vi "ViperHawk Get Diagnostic Data.vi"(6 "Command":enum16{"9E", "9F"}(ring), 10 "Hex String In":string, 11 "Diagnostic":T1) -> (3 "Diagnostic Data Output":T1)   [LabVIEW 2016]
uses:
  Type Definitions/ViperHawk/ViperHawk Diagnostic Data.ctl
  Utility/LabVIEW GEA2 Toolkit v1.0.0.0/library/GEA2_Toolkit.lvlib
  <vilib>/ptbypt/NI_PtbyPt.lvlib
panel:
  out "String":string
  out "Cycle Number":u32
  out "Hex Array Out":u8[](array[numeric]) format="%.0x"
  # "00 00 BF 27 01 B7 00 7B 00 00 00 00 00 00 00 00 14 64 0F 01 01 00 00 81"
  # "9F\n01 02"
  # "9F"
  # "01 02 03 63 00 00 04 00 04 05 00 04 02 00 00 00 00 00 00 00 00 01 00 00 00 00"
  # "9E"
  # "00 00 AA E1 03 65 03 E1 00 00 00 00 00 00 00 00 14 64 0F 01 04 00 00 40"
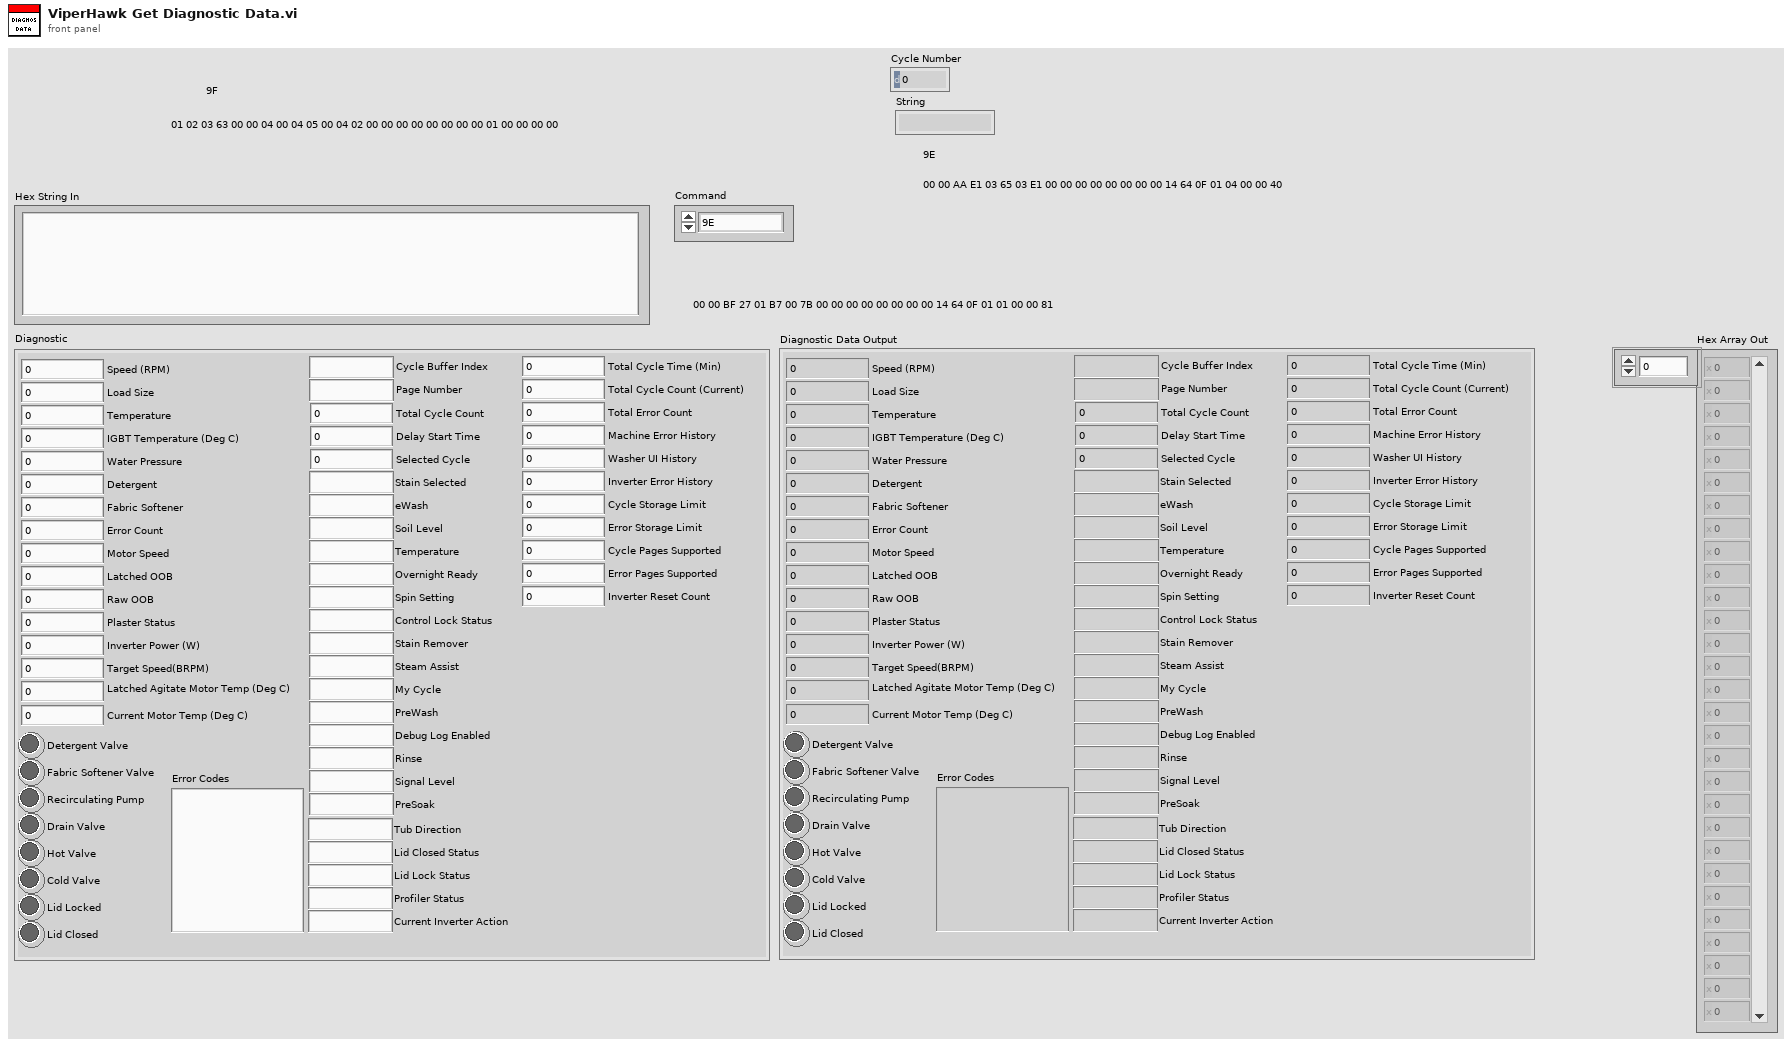
[diagram p1: front panel]
types:
  T1 = typedef "ViperHawk Diagnostic Data.ctl" = cluster{"Speed (RPM)":u32, "Load Size":u32, "Temperature":u32, "Water Pressure":dbl, "Detergent":u32, "Fabric Softener":u32, "Tub Direction":string, "Detergent Valve":bool, "Fabric Softener Valve":bool, "Recirculating Pump":bool, "Drain Valve":bool, "Hot Valve":bool, "Cold Valve":bool, "Lid Closed Status":string, "Lid Lock Status":string, "Error Count":u32, "IGBT Temperature (Deg C)":u32, "Motor Speed":u32, "Latched OOB":u32, "Raw OOB":u32, "Plaster Status":u32, "Inverter Power (W)":u32, "Target Speed(BRPM)":u32, "Latched Agitate Motor Temp (Deg C)":u32, "Current Motor Temp (Deg C)":u32, "Profiler Status":string, "Current Inverter Action":string, "Error Codes":string, "Lid Locked":bool, "Lid Closed":bool, "9E Diagnostic Data":cluster{"Total Cycle Time (Min)":u32, "Total Cycle Count (Current)":u16, "Total Error Count":u16, "Machine Error History":u32, "Washer UI History":u32, "Inverter Error History":u32, "Cycle Storage Limit":u8, "Error Storage Limit":u8, "Cycle Pages Supported":u8, "Error Pages Supported":u8, "Inverter Reset Count":u16}, "9F Diagnostic Data":cluster{"Cycle Buffer Index":string, "Page Number":string, "Total Cycle Count":u32, "Delay Start Time":u32, "Stain Selected":string, "Selected Cycle":u32, "eWash":string, "Soil Level":string, "Temperature":string, "Overnight Ready":string, "Spin Setting":string, "Control Lock Status":string, "Stain Remover":string, "Steam Assist":string, "My Cycle":string, "PreWash":string, "Debug Log Enabled":string, "Rinse":string, "Signal Level":string, "PreSoak":string}}
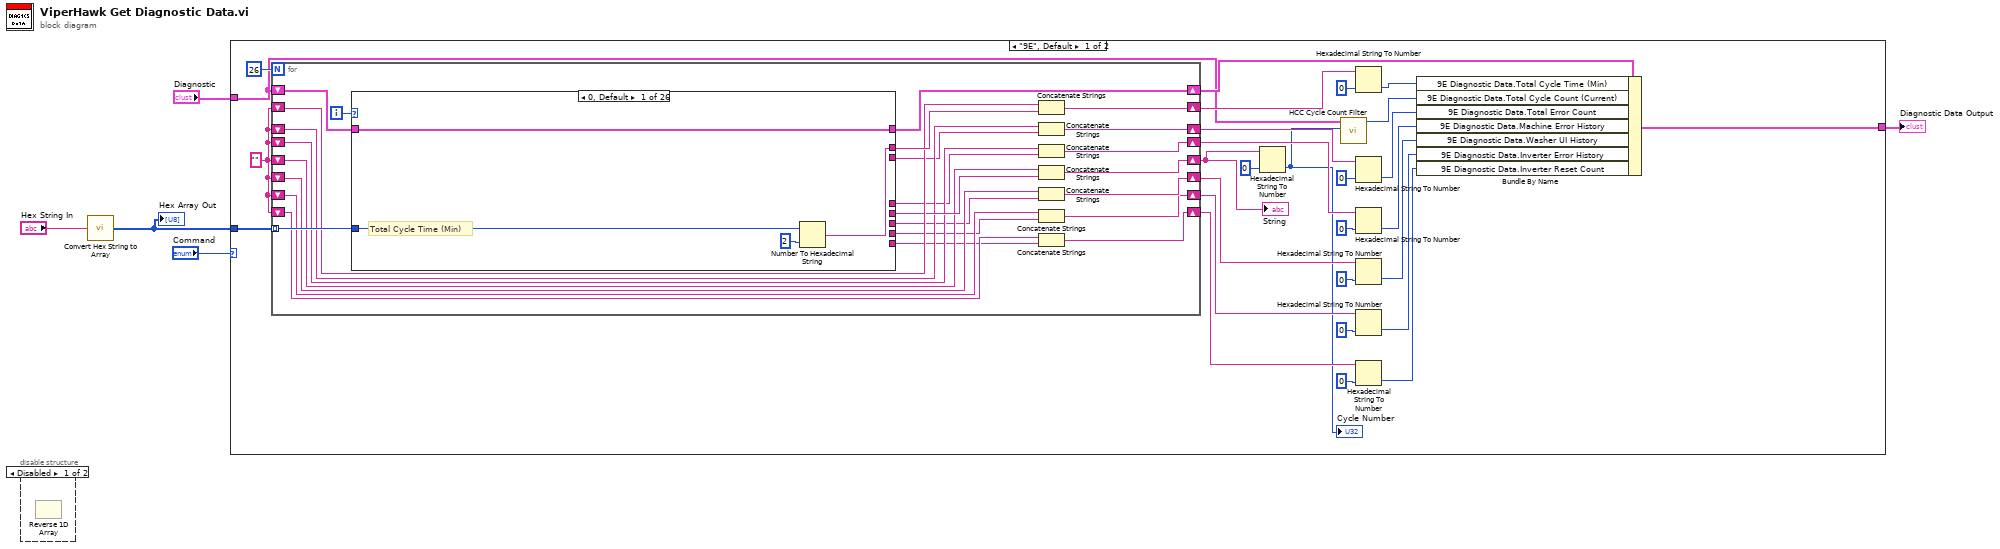
[diagram p0: block diagram]
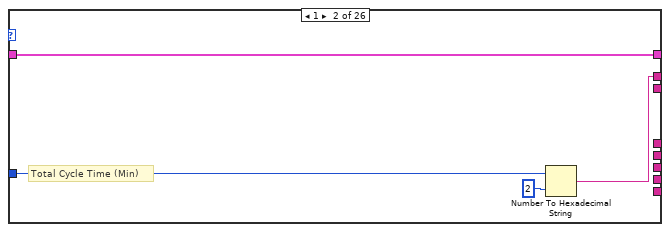
[diagram p3: hidden frame]
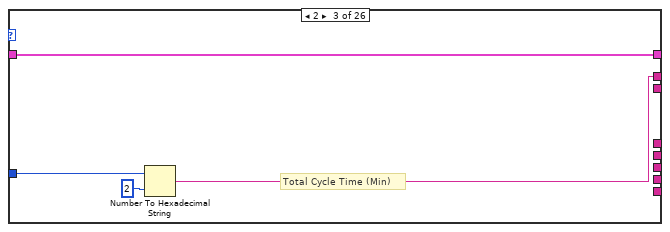
[diagram p4: hidden frame]
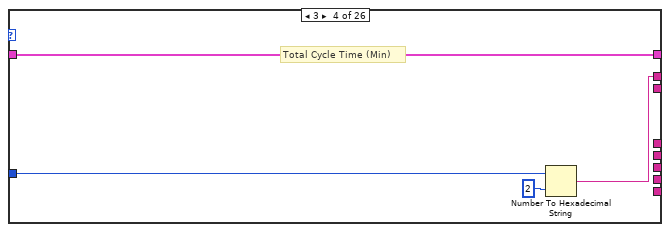
[diagram p5: hidden frame]
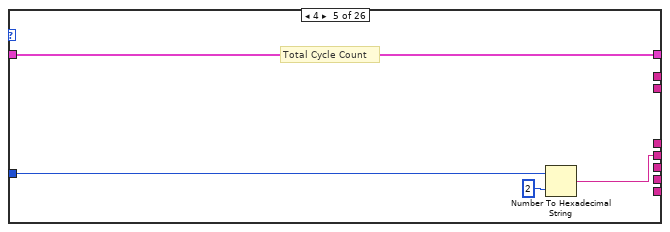
[diagram p6: hidden frame]
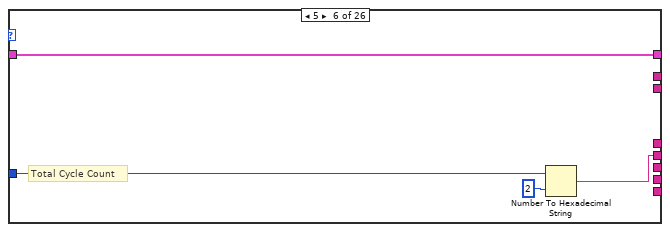
[diagram p7: hidden frame]
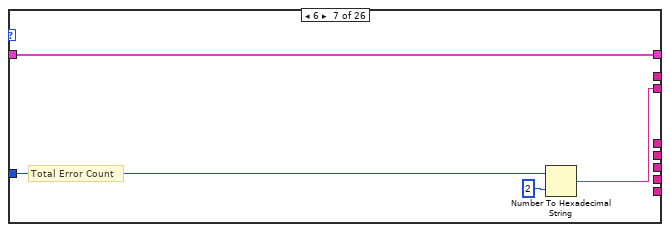
[diagram p8: hidden frame]
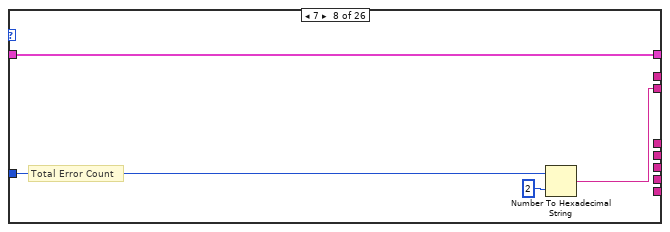
[diagram p9: hidden frame]
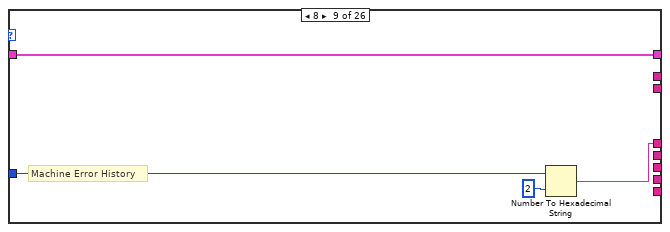
[diagram p10: hidden frame]
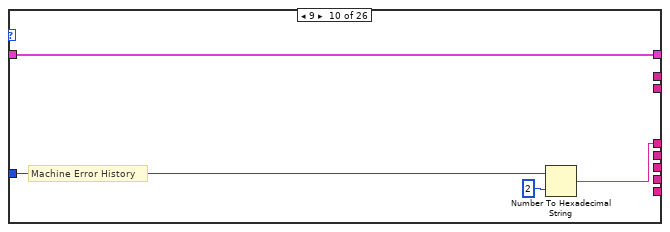
[diagram p11: hidden frame]
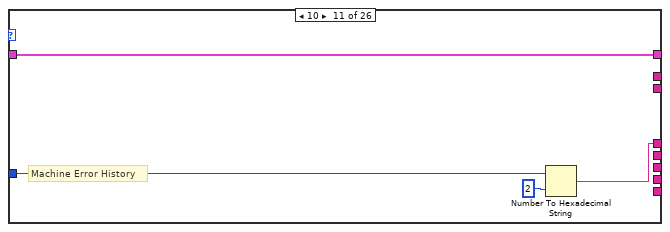
[diagram p12: hidden frame]
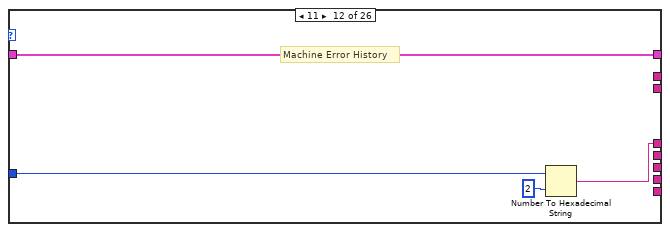
[diagram p13: hidden frame]
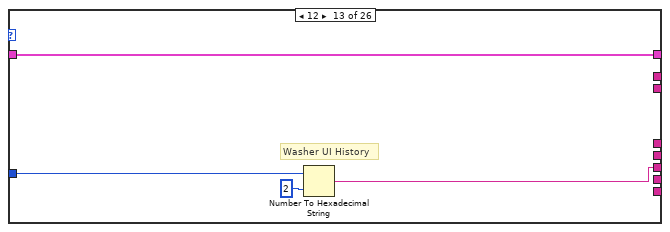
[diagram p14: hidden frame]
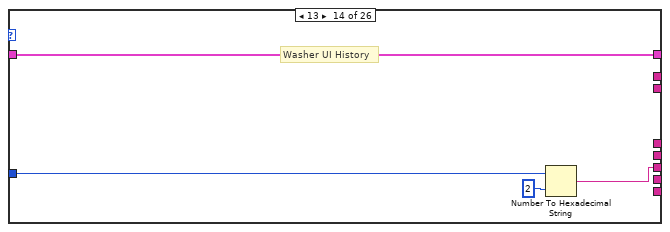
[diagram p15: hidden frame]
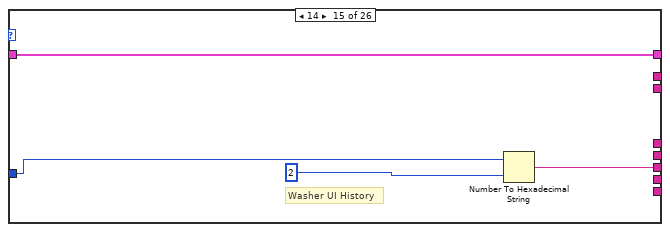
[diagram p16: hidden frame]
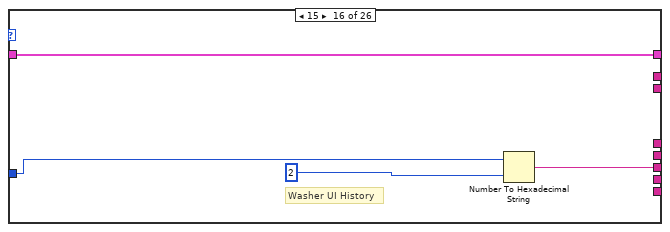
[diagram p17: hidden frame]
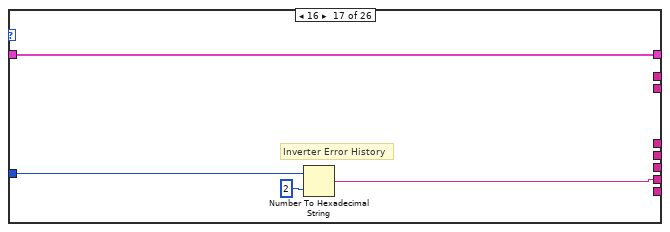
[diagram p18: hidden frame]
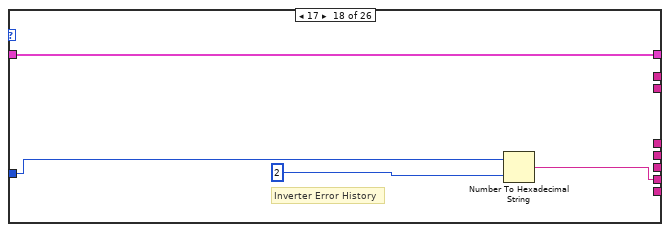
[diagram p19: hidden frame]
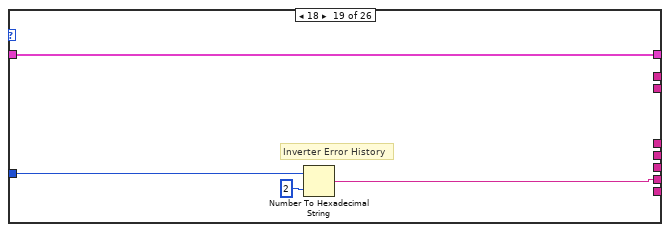
[diagram p20: hidden frame]
diagram:
  n1 = disable-structure shown="Disabled" {
    frame Disabled {
      n2 = Reverse 1D Array() -> ()  [unwired: 1 in, 1 out]
    }
    frame Enabled {
    }
  }
  n3 = call "Convert Hex String to Array.vi"("Hex String In"="Hex String In") -> ("Hex Array Out"=w1:u8[])  [unwired: 14 in]
  "Hex Array Out" <- w1
  n4 = case shown="\"9E\", Default" "Command" {
    tunnel: w1 -> [w30 w164]
    tunnel: "Diagnostic" -> [w6 w163]
    tunnel: [w29 w161] -> w3
    frame "9E", Default {
      w28 = ""
      n5 = for {
        N: 26 -> [_]
        tunnel: w30 -> [w58] mode=indexing
        shift-right: [w49] -> w32
        shift-left: w28 -> [w56]
        shift-right: [w54] -> w33
        shift-left: w28 -> [w51]
        shift-right: [w52] -> w9
        shift-left: w6 -> [w53]
        shift-right: [w48] -> w21
        shift-left: w28 -> [w43]
        shift-right: [w47] -> w25
        shift-left: w28 -> [w42]
        shift-right: [w46] -> w17
        shift-left: w28 -> [w41]
        shift-right: [w45] -> w19
        shift-left: w28 -> [w40]
        shift-right: [w44] -> w23
        shift-left: w28 -> [w39]
        i -> [w50]
        n6 = case shown="0, Default" w50 {
          tunnel: w58 -> [w60 w65 w68 w72 w78 w82 w84 w88 w92 w96 w100 w104 w108 w112 w116 w120 w124 w128 w132 w136 w139 w142 w145 w148 w152 w156]
          tunnel: [w59 w64 w67 w71 _ _ _ _ _ _ _ _ _ _ _ _ _ _ _ _ _ _ _ _ _ _] -> w57
          tunnel: [_ _ _ _ w75 w79 _ _ _ _ _ _ _ _ _ _ _ _ _ _ _ _ _ _ _ _] -> w55
          tunnel: w53 -> [w62 w63 w70 w74 w77 w81 w86 w90 w94 w98 w102 w106 w110 w114 w118 w122 w126 w130 w134 w138 w141 w144 w147 w150 w154 w158]
          tunnel: [w62 w63 w70 w74 w77 w81 w86 w90 w94 w98 w102 w106 w110 w114 w118 w122 w126 w130 w134 w138 w140 w143 w146 w149 w154 w158] -> w52
          tunnel: [_ _ _ _ _ _ w83 w87 _ _ _ _ _ _ _ _ _ _ _ _ _ _ _ _ _ _] -> w38
          tunnel: [_ _ _ _ _ _ _ _ w91 w95 w99 w103 _ _ _ _ _ _ _ _ _ _ _ _ _ _] -> w37
          tunnel: [_ _ _ _ _ _ _ _ _ _ _ _ w107 w111 w115 w119 _ _ _ _ _ _ _ _ _ _] -> w36
          tunnel: [_ _ _ _ _ _ _ _ _ _ _ _ _ _ _ _ w123 w127 w131 w135 _ _ _ _ _ _] -> w35
          tunnel: [_ _ _ _ _ _ _ _ _ _ _ _ _ _ _ _ _ _ _ _ _ _ _ _ w151 w155] -> w34
          frame 0, Default {
            # "Total Cycle Time (Min)"
            n7 = Number To Hexadecimal String(1:i16 2 ("width (-)"), 2:w60) -> (0:w59:string)
          }
          frame 1 {
            # "Total Cycle Time (Min)"
            n8 = Number To Hexadecimal String(1:i16 2 ("width (-)"), 2:w65) -> (0:w64:string)
          }
          frame 2 {
            # "Total Cycle Time (Min)"
            n9 = Number To Hexadecimal String(1:i16 2 ("width (-)"), 2:w68) -> (0:w67:string)
          }
          frame 3 {
            # "Total Cycle Time (Min)"
            n10 = Number To Hexadecimal String(1:i16 2 ("width (-)"), 2:w72) -> (0:w71:string)
          }
          frame 4 {
            # "Total Cycle Count"
            n11 = Number To Hexadecimal String(1:i16 2 ("width (-)"), 2:w78) -> (0:w75:string)
          }
          frame 5 {
            # "Total Cycle Count"
            n12 = Number To Hexadecimal String(1:i16 2 ("width (-)"), 2:w82) -> (0:w79:string)
          }
          frame 6 {
            # "Total Error Count"
            n13 = Number To Hexadecimal String(1:i16 2 ("width (-)"), 2:w84) -> (0:w83:string)
          }
          frame 7 {
            # "Total Error Count"
            n14 = Number To Hexadecimal String(1:i16 2 ("width (-)"), 2:w88) -> (0:w87:string)
          }
          frame 8 {
            # "Machine Error History"
            n15 = Number To Hexadecimal String(1:i16 2 ("width (-)"), 2:w92) -> (0:w91:string)
          }
          frame 9 {
            # "Machine Error History"
            n16 = Number To Hexadecimal String(1:i16 2 ("width (-)"), 2:w96) -> (0:w95:string)
          }
          frame 10 {
            # "Machine Error History"
            n17 = Number To Hexadecimal String(1:i16 2 ("width (-)"), 2:w100) -> (0:w99:string)
          }
          frame 11 {
            # "Machine Error History"
            n18 = Number To Hexadecimal String(1:i16 2 ("width (-)"), 2:w104) -> (0:w103:string)
          }
          frame 12 {
            # "Washer UI History"
            n19 = Number To Hexadecimal String(1:i16 2 ("width (-)"), 2:w108) -> (0:w107:string)
          }
          frame 13 {
            # "Washer UI History"
            n20 = Number To Hexadecimal String(1:i16 2 ("width (-)"), 2:w112) -> (0:w111:string)
          }
          frame 14 {
            # "Washer UI History"
            n21 = Number To Hexadecimal String(1:i16 2 ("width (-)"), 2:w116) -> (0:w115:string)
          }
          frame 15 {
            # "Washer UI History"
            n22 = Number To Hexadecimal String(1:i16 2 ("width (-)"), 2:w120) -> (0:w119:string)
          }
          frame 16 {
            # "Inverter Error History"
            n23 = Number To Hexadecimal String(1:i16 2 ("width (-)"), 2:w124) -> (0:w123:string)
          }
          frame 17 {
            # "Inverter Error History"
            n24 = Number To Hexadecimal String(1:i16 2 ("width (-)"), 2:w128) -> (0:w127:string)
          }
          frame 18 {
            # "Inverter Error History"
            n25 = Number To Hexadecimal String(1:i16 2 ("width (-)"), 2:w132) -> (0:w131:string)
          }
          frame 19 {
            # "Inverter Error History"
            n26 = Number To Hexadecimal String(1:i16 2 ("width (-)"), 2:w136) -> (0:w135:string)
          }
          frame 20 {
            n27 = Bundle By Name(cluster=w141, "9E Diagnostic Data.Cycle Storage Limit"=w139) -> (w140:T1)
          }
          frame 21 {
            n28 = Bundle By Name(cluster=w144, "9E Diagnostic Data.Error Storage Limit"=w142) -> (w143:T1)
          }
          frame 22 {
            n29 = Bundle By Name(cluster=w147, "9E Diagnostic Data.Cycle Pages Supported"=w145) -> (w146:T1)
          }
          frame 23 {
            n30 = Bundle By Name(cluster=w150, "9E Diagnostic Data.Error Pages Supported"=w148) -> (w149:T1)
          }
          frame 24 {
            # "Inverter Reset Count"
            n31 = Number To Hexadecimal String(1:i16 2 ("width (-)"), 2:w152) -> (0:w151:string)
          }
          frame 25 {
            # "Inverter Reset Count"
            n32 = Number To Hexadecimal String(1:i16 2 ("width (-)"), 2:w156) -> (0:w155:string)
          }
        }
        n33 = Concatenate Strings(w56, w57) -> (w49:string)
        n34 = Concatenate Strings(w43, w38) -> (w48:string)
        n35 = Concatenate Strings(w39, w37) -> (w44:string)
        n36 = Concatenate Strings(w51, w55) -> (w54:string)
        n37 = Concatenate Strings(w42, w36) -> (w47:string)
        n38 = Concatenate Strings(w41, w35) -> (w46:string)
        n39 = Concatenate Strings(w40, w34) -> (w45:string)
      }
      "String" <- w33
      n40 = Hexadecimal String To Number(string=w33, default (0uL)=u16 0 ("default (0 U32)")) -> (number=w8:u16)  [unwired: 1 in, 1 out]
      "Cycle Number" <- w8
      n41 = call "HCC Cycle Count Filter.vi"("Incoming Cycle Count"=w8, "Diagnostic"=w6) -> ("Filtered Cycle Count"=w7:u16)  [unwired: 7 in, 2 out]
      n42 = Hexadecimal String To Number(string=w32, default (0uL)=u32 0 ("default (0 U32)")) -> (number=w26:u32)  [unwired: 1 in, 1 out]
      n43 = Hexadecimal String To Number(string=w21, default (0uL)=u16 0 ("default (0 U32)")) -> (number=w20:u16)  [unwired: 1 in, 1 out]
      n44 = Hexadecimal String To Number(string=w23, default (0uL)=u32 0 ("default (0 U32)")) -> (number=w22:u32)  [unwired: 1 in, 1 out]
      n45 = Hexadecimal String To Number(string=w25, default (0uL)=u32 0 ("default (0 U32)")) -> (number=w24:u32)  [unwired: 1 in, 1 out]
      n46 = Hexadecimal String To Number(string=w17, default (0uL)=u32 0 ("default (0 U32)")) -> (number=w16:u32)  [unwired: 1 in, 1 out]
      n47 = Hexadecimal String To Number(string=w19, default (0uL)=u16 0 ("default (0 U32)")) -> (number=w18:u16)  [unwired: 1 in, 1 out]
      n48 = Bundle By Name(cluster=w9, "9E Diagnostic Data.Total Cycle Time (Min)"=w26, "9E Diagnostic Data.Total Cycle Count (Current)"=w7, "9E Diagnostic Data.Total Error Count"=w20, "9E Diagnostic Data.Machine Error History"=w22, "9E Diagnostic Data.Washer UI History"=w24, "9E Diagnostic Data.Inverter Error History"=w16, "9E Diagnostic Data.Inverter Reset Count"=w18) -> (w29:T1)
    }
    frame "9F" {
      w167 = ""
      n49 = for {
        N: 22 -> [_]
        tunnel: w164 -> [w179] mode=indexing
        shift-right: [w176] -> w168
        shift-left: w167 -> [w177]
        shift-right: [w174] -> w169
        shift-left: w167 -> [w171]
        shift-right: [w172] -> w166
        shift-left: w163 -> [w173]
        i -> [w170]
        n50 = case shown="15" w170 {
          tunnel: w179 -> [w181 w188 w194 w198 w204 w208 w210 w215 w219 w225 w234 w244 w250 w259 w265 w271 w277 w283 w289 w295 w304 w313]
          tunnel: [w184 _ _ _ w203 w207 _ _ _ _ _ _ _ _ _ _ _ _ _ _ _ _] -> w178
          tunnel: [w184 _ _ _ _ _ _ _ _ _ _ _ _ _ _ _ _ _ _ _ _ _] -> _
          tunnel: [w184 _ w193 w197 _ _ _ _ _ _ _ _ _ _ _ _ _ _ _ _ _ _] -> w175
          tunnel: w173 -> [w183 w190 w196 w200 w202 w206 w212 w217 w221 w227 w236 w246 w252 w261 w267 w273 w279 w285 w291 w297 w306 w315]
          tunnel: [w182 w189 w196 w200 w202 w206 w211 w216 w220 w226 w235 w245 w251 w260 w266 w272 w278 w284 w290 w296 w305 w314] -> w172
          frame 0, Default {
            w184 = ""
            n51 = case shown="1, Default" w181 {
              tunnel: ["Active cycle" "2nd most recent"] -> w180
              frame 1, Default {
              }
              frame 2 {
              }
            }
            n52 = Bundle By Name(cluster=w183, "9F Diagnostic Data.Cycle Buffer Index"=w180) -> (w182:T1)
          }
          frame 1 {
            n53 = case shown="1, Default" w188 {
              tunnel: [" Start user options" "EOC options"] -> w187
              frame 1, Default {
              }
              frame 2 {
              }
            }
            n54 = Bundle By Name(cluster=w190, "9F Diagnostic Data.Page Number"=w187) -> (w189:T1)
          }
          frame 2 {
            # "Cycle Count"
            n55 = Number To Hexadecimal String(1:i16 2 ("width (-)"), 2:w194) -> (0:w193:string)
          }
          frame 3 {
            # "Cycle Count"
            n56 = Number To Hexadecimal String(1:i16 2 ("width (-)"), 2:w198) -> (0:w197:string)
          }
          frame 4 {
            # "Delay Start Time"
            n57 = Number To Hexadecimal String(1:i16 2 ("width (-)"), 2:w204) -> (0:w203:string)
          }
          frame 5 {
            # "Delay Start Time"
            n58 = Number To Hexadecimal String(1:i16 2 ("width (-)"), 2:w208) -> (0:w207:string)
          }
          frame 6 {
            n59 = case shown="1" w210 {
              tunnel: ["Off" "On"] -> w209
              frame 0, Default {
              }
              frame 1 {
              }
            }
            n60 = Bundle By Name(cluster=w212, "9F Diagnostic Data.Stain Selected"=w209) -> (w211:T1)
          }
          frame 7 {
            n61 = Bundle By Name(cluster=w217, "9F Diagnostic Data.Selected Cycle"=w215) -> (w216:T1)
          }
          frame 8 {
            n62 = case shown="1" w219 {
              tunnel: ["Off" "On"] -> w218
              frame 0, Default {
              }
              frame 1 {
              }
            }
            n63 = Bundle By Name(cluster=w221, "9F Diagnostic Data.eWash"=w218) -> (w220:T1)
          }
          frame 9 {
            n64 = case shown="4" w225 {
              tunnel: ["Extra Light" "Light" "Normal" "Heavy" "Extra Heavy"] -> w224
              frame 0, Default {
              }
              frame 1 {
              }
              frame 2 {
              }
              frame 3 {
              }
              frame 4 {
              }
            }
            n65 = Bundle By Name(cluster=w227, "9F Diagnostic Data.Soil Level"=w224) -> (w226:T1)
          }
          frame 10 {
            n66 = case shown="5" w234 {
              tunnel: ["Tap Cold" "Cold" "Warm" "Hot" "Extra Hot" "Extra Hot"] -> w233
              frame 0, Default {
              }
              frame 1 {
              }
              frame 2 {
              }
              frame 3 {
              }
              frame 4 {
              }
              frame 5 {
              }
            }
            n67 = Bundle By Name(cluster=w236, "9F Diagnostic Data.Temperature"=w233) -> (w235:T1)
          }
          frame 11 {
            n68 = case shown="0, Default" w244 {
              tunnel: ["Off" "On"] -> w243
              frame 0, Default {
              }
              frame 1 {
              }
            }
            n69 = Bundle By Name(cluster=w246, "9F Diagnostic Data.Overnight Ready"=w243) -> (w245:T1)
          }
          frame 12 {
            n70 = case shown="4" w250 {
              tunnel: ["No Spin" "Low" "Medium" "High" "Extra High"] -> w249
              frame 0, Default {
              }
              frame 1 {
              }
              frame 2 {
              }
              frame 3 {
              }
              frame 4 {
              }
            }
            n71 = Bundle By Name(cluster=w252, "9F Diagnostic Data.Spin Setting"=w249) -> (w251:T1)
          }
          frame 13 {
            n72 = case shown="0, Default" w259 {
              tunnel: ["Off" "On"] -> w258
              frame 0, Default {
              }
              frame 1 {
              }
            }
            n73 = Bundle By Name(cluster=w261, "9F Diagnostic Data.Control Lock Status"=w258) -> (w260:T1)
          }
          frame 14 {
            n74 = case shown="1" w265 {
              tunnel: ["Off" "On"] -> w264
              frame 0, Default {
              }
              frame 1 {
              }
            }
            n75 = Bundle By Name(cluster=w267, "9F Diagnostic Data.Stain Remover"=w264) -> (w266:T1)
          }
          frame 15 {
            n76 = case shown="1" w271 {
              tunnel: ["Off" "On"] -> w270
              frame 0, Default {
              }
              frame 1 {
              }
            }
            n77 = Bundle By Name(cluster=w273, "9F Diagnostic Data.Steam Assist"=w270) -> (w272:T1)
          }
          frame 16 {
            n78 = case shown="1" w277 {
              tunnel: ["Off" "On"] -> w276
              frame 0, Default {
              }
              frame 1 {
              }
            }
            n79 = Bundle By Name(cluster=w279, "9F Diagnostic Data.My Cycle"=w276) -> (w278:T1)
          }
          frame 17 {
            n80 = case shown="1" w283 {
              tunnel: ["Off" "On"] -> w282
              frame 0, Default {
              }
              frame 1 {
              }
            }
            n81 = Bundle By Name(cluster=w285, "9F Diagnostic Data.PreWash"=w282) -> (w284:T1)
          }
          frame 18 {
            n82 = case shown="1" w289 {
              tunnel: ["Off" "On"] -> w288
              frame 0, Default {
              }
              frame 1 {
              }
            }
            n83 = Bundle By Name(cluster=w291, "9F Diagnostic Data.Debug Log Enabled"=w288) -> (w290:T1)
          }
          frame 19 {
            n84 = case shown="4" w295 {
              tunnel: ["Off" "Normal" "Extra" "Max" "4"] -> w294
              frame 0, Default {
              }
              frame 1 {
              }
              frame 2 {
              }
              frame 3 {
              }
              frame 4 {
              }
            }
            n85 = Bundle By Name(cluster=w297, "9F Diagnostic Data.Rinse"=w294) -> (w296:T1)
          }
          frame 20 {
            n86 = case shown="4" w304 {
              tunnel: ["Off" "Low" "Medium" "High" "4"] -> w303
              frame 0, Default {
              }
              frame 1 {
              }
              frame 2 {
              }
              frame 3 {
              }
              frame 4 {
              }
            }
            n87 = Bundle By Name(cluster=w306, "9F Diagnostic Data.Signal Level"=w303) -> (w305:T1)
          }
          frame 21 {
            n88 = case shown="10" w313 {
              tunnel: ["Off" "30 Min" "1 Hr" "1:30 Hr" "2 Hr" "2:30 Hr" "3 Hr" "3:30 Hr" "4 Hr" "4:30 Hr" "5 Hr" "5:30 Hr" "6 Hr" "6:30 Hr" "7 Hr" "7:30 Hr" "8 Hr"] -> w312
              frame 0, Default {
              }
              frame 1 {
              }
              frame 2 {
              }
              frame 3 {
              }
              frame 4 {
              }
              frame 5 {
              }
              frame 6 {
              }
              frame 7 {
              }
              frame 8 {
              }
              frame 9 {
              }
              frame 10 {
              }
              frame 11 {
              }
              frame 12 {
              }
              frame 13 {
              }
              frame 14 {
              }
              frame 15 {
              }
              frame 16 {
              }
            }
            n89 = Bundle By Name(cluster=w315, "9F Diagnostic Data.PreSoak"=w312) -> (w314:T1)
          }
        }
        n90 = Concatenate Strings(w171, w175) -> (w174:string)
        n91 = Concatenate Strings(w177, w178) -> (w176:string)
      }
      n92 = Hexadecimal String To Number(string=w169) -> (number=w160:u32)  [unwired: 2 in, 1 out]
      n93 = Hexadecimal String To Number(string=w168) -> (number=w165:u32)  [unwired: 2 in, 1 out]
      n94 = call <vilib>:"Median Filter PtByPt.vi"("x"=w160) -> ("Filtered x"=w159:dbl)  [unwired: 3 in, 1 out]
      n95 = Bundle By Name(cluster=w166, "9F Diagnostic Data.Total Cycle Count"=w159, "9F Diagnostic Data.Delay Start Time"=w165) -> (w161:T1)
    }
  }
  "Diagnostic Data Output" <- w3
